vi "Build num command substring.vi"(2 "Num 1":dbl[](array[numeric]) format="%.6f", 3 "Num 2":dbl[](array[numeric]) format="%.6f", 4 "No. of digits":i16=4) -> (14 "Command substring":string)   [LabVIEW 2026]
doc: "This VI builds a command substring by combining Num 1, Space and Num 2. No. of digits is the number of digits after the decimal point in the Num 1/2 value(s) that will be sent.\nExample: For Num 1 = 1.24; 3.25456, Num 2 = 5.0; 7.4321 and No. of digits = 3 the resulting string is \"Space1.240Space5.000Space3.255Space7.432\"."
panel:
  # "This vi builds a command substring by combining Num 1, Space and Num 2."
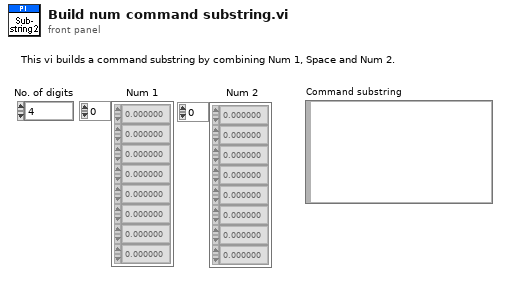
[diagram p1: front panel]
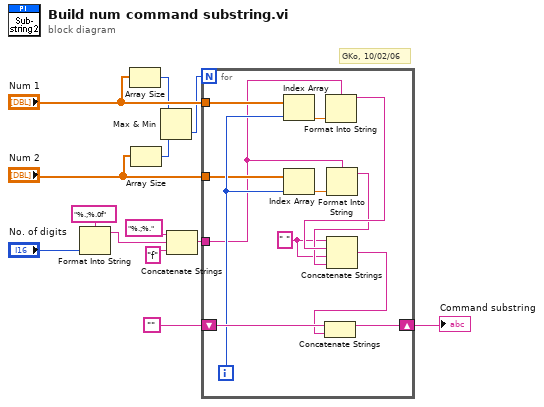
[diagram p0: block diagram]
diagram:
  # "GKo, 10/02/06"
  n1 = Format Into String(format string="%.;%.0f" ("Format String"), "No. of digits") -> (resulting string=w3:string)  [unwired: 2 in, 1 out]
  n2 = Array Size(array="Num 1") -> (size(s)=w8:i32)
  n3 = Array Size(array="Num 2") -> (size(s)=w9:i32)
  n4 = Max & Min(x=w8, y=w9) -> (min(x,y)=w7:i32)  [unwired: 1 out]
  n5 = Concatenate Strings("%.;%." ("Format String"), w3, "f" ("Format String")) -> (w1:string)
  n6 = for {
    N: w7 -> [_]
    shift-right: [w24] -> w12
    shift-left: "" -> [w25]
    tunnel: "Num 2" -> [w21]
    tunnel: w1 -> [w16]
    tunnel: "Num 1" -> [w20]
    i -> [w22]
    w14 = " " ("Substring")
    n7 = Index Array(array=w20, index=w22) -> (element=w18:dbl)
    n8 = Index Array(array=w21, index=w22) -> (element=w19:dbl)
    n9 = Format Into String(format string=w16, w18) -> (resulting string=w17:string)  [unwired: 2 in, 1 out]
    n10 = Format Into String(format string=w16, w19) -> (resulting string=w15:string)  [unwired: 2 in, 1 out]
    n11 = Concatenate Strings(w14, w17, w14, w15) -> (w23:string)
    n12 = Concatenate Strings(w25, w23) -> (w24:string)
  }
  "Command substring" <- w12
